vi "4Pi OIA - Norm Cross Corr.vi"(0 "Image 01":u16[][](array[numeric]), 11 "Image 02":u16[][](array[numeric]), 13 "Half Shift":i32=7) -> (8 "Norm Cross Corr Result":dbl[][](array[numeric]))   [LabVIEW 2016]
uses:
  Wide Field Drift Correction/WFDC DLL and Testing/Visual Studio NCC Max Shift DLL/x64/Release/VSmaxShiftNCC.dll
panel:
  out "Norm Cross Corr Image":dbl[][](graph)
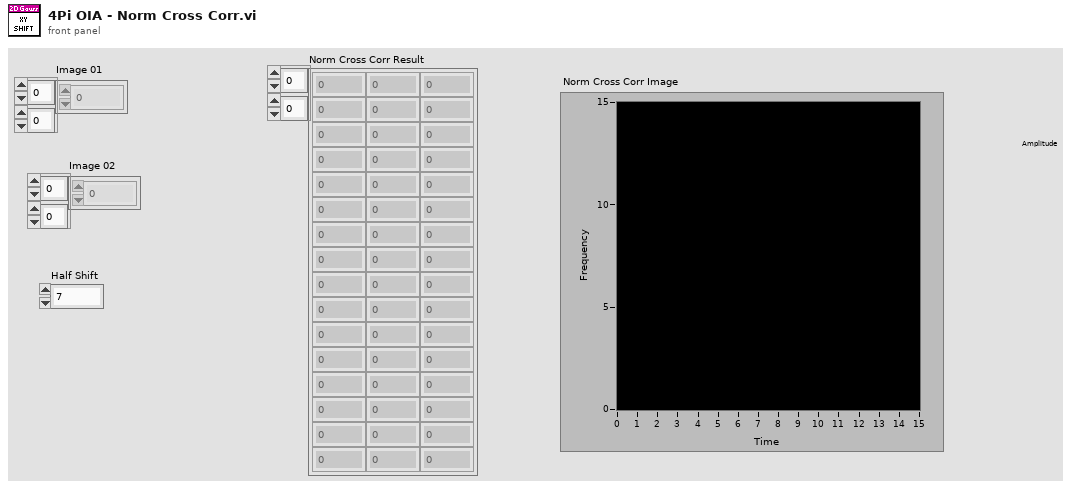
[diagram p1: front panel]
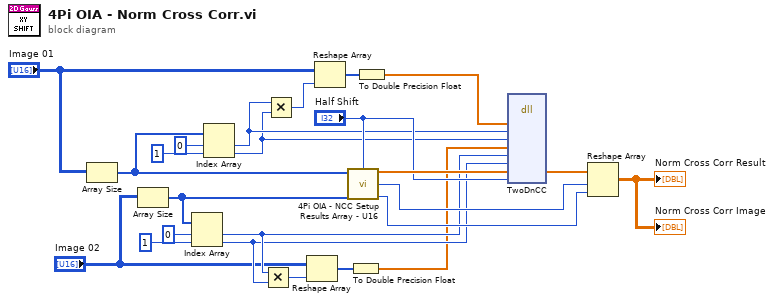
[diagram p0: block diagram]
diagram:
  n1 = Array Size(array="Image 01") -> (size(s)=w8:i32[])
  n2 = Array Size(array="Image 02") -> (size(s)=w18:i32[])
  n3 = Index Array(array=w18, index #1=0 ("index"), index #2=1 ("index")) -> (element #1=w15:i32, element #2=w14:i32)
  n4 = Index Array(array=w8, index #1=0 ("index"), index #2=1 ("index")) -> (element #1=w5:i32, element #2=w4:i32)
  n5 = Multiply(x=w15, y=w14) -> (x*y=w13:i32)
  n6 = Multiply(x=w5, y=w4) -> (x*y=w3:i32)
  n7 = Reshape Array("Image 02", w13) -> (w12:u16[])
  n8 = Reshape Array("Image 01", w3) -> (w7:u16[])
  n9 = call "4Pi OIA - NCC Setup Results Array - U16.vi"("Image 01 Size"=w8, "Half Shift"="Half Shift", "Image 02 Size"=w18) -> ("NCC Results Array"=w23:dbl[], "Result Rows"=w20:i32, "Result Columns"=w21:i32)  [unwired: 10 in]
  n10 = To Double Precision Float(number=w12) -> (double precision float=w11:dbl[])
  n11 = To Double Precision Float(number=w7) -> (double precision float=w6:dbl[])
  n12 = dll-call lib="C:/Users/George Sirinakis/Documents/Microscope-Control/Microscope Modules/Wide Field Drift Correction/WFDC DLL and Testing/Visual Studio NCC Max Shift DLL/x64/Release/VSmaxShiftNCC.dll" fn="TwoDnCC"("im01"=w6, "im01rowSize"=w5, "im01colSize"=w4, "im02"=w11, "im02rowSize"=w15, "im02ColSize"=w14, "theResult"=w23, "halfShift"="Half Shift") -> ("theResult"=w22:dbl[])  [unwired: 11 in, 2 out]
  n13 = Reshape Array(w22, w20, w21) -> (→"Norm Cross Corr Image" →"Norm Cross Corr Result":dbl[][])
